vi "Adjust Text Label.vi"(8 "error in (no error)":errorcluster, 11 "Label Ref":refnum<vi>) -> (0 "error out":errorcluster, 2 "Changed?":bool)   [LabVIEW 2020]
uses:
  <vilib>/Utility/miscctls.llb/LVSelectionTypeDef.ctl
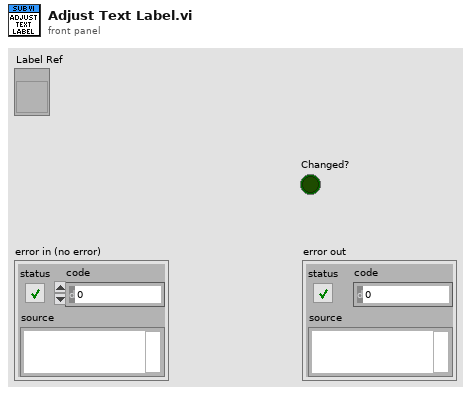
[diagram p1: front panel]
types:
  T1 = typedef "LVSelectionTypeDef.ctl" = cluster{"Selection Start":u32, "Selection End":u32}
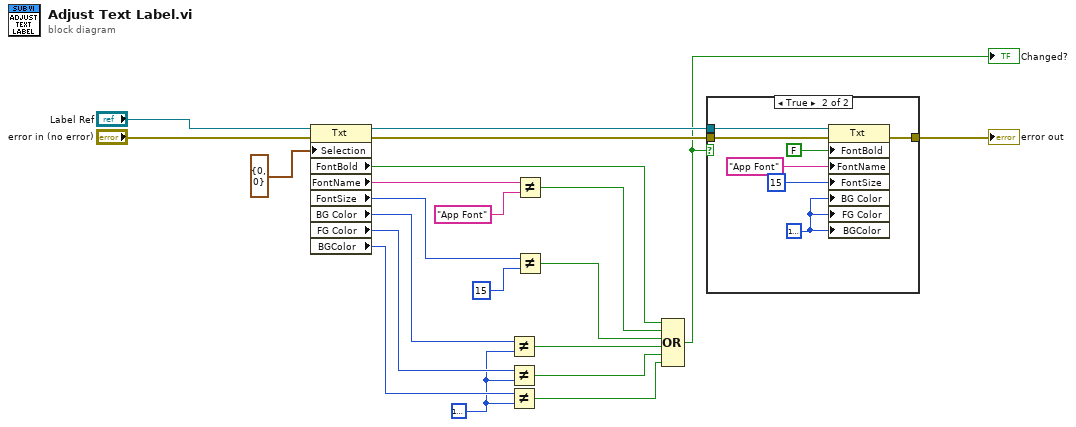
[diagram p0: block diagram]
diagram:
  w11 = u32 16777216
  n1 = property class="Txt"(reference="Label Ref", error in="error in (no error)", "Selection"=T1 {"Selection Start"=0, "Selection End"=0} ("Label.Selection")) -> (reference out=w21:refnum<vi>, error out=w20:errorcluster, "FontBold"=w15:bool, "FontName"=w6:string, "FontSize"=w4:u32, "BG Color"=w18:u32, "FG Color"=w17:u32, "BGColor"=w12:u32)
  n2 = Not Equal?(x=w18, y=w11) -> (x != y?=w19:bool)
  n3 = Not Equal?(x=w17, y=w11) -> (x != y?=w16:bool)
  n4 = Not Equal?(x=w12, y=w11) -> (x != y?=w10:bool)
  n5 = Not Equal?(x=w6, y="App Font") -> (x != y?=w1:bool)
  n6 = Not Equal?(x=w4, y=u32 15) -> (x != y?=w2:bool)
  n7 = Compound Arithmetic op=OR(w15, w1, w2, w19, w16, w10) -> (w14:bool)
  "Changed?" <- w14
  n8 = case shown="True" w14 {
    tunnel: w21 -> [_ w29]
    tunnel: w20 -> [w22 w28]
    tunnel: [w22 w26] -> w8
    frame False {
    }
    frame True {
      w25 = u32 16777216
      n9 = property class="Txt"(reference=w29, error in=w28, "FontBold"=FALSE ("AutoSize To Fit Contents?"), "FontName"="App Font" ("y"), "FontSize"=u32 15 ("y"), "BG Color"=w25, "FG Color"=w25, "BGColor"=w25) -> (error out=w26:errorcluster)  [unwired: 1 out]
    }
  }
  "error out" <- w8
